vi "Packing_Barcode.vi"(7 "timeout ms":i32, 8 "error in (no error)":errorcluster, 9 "data in":string, 10 "PRINT":u16, 11 "IP":string) -> (0 "error out":errorcluster)   [LabVIEW 2017]
panel:
  # "Packing Barcode Print"
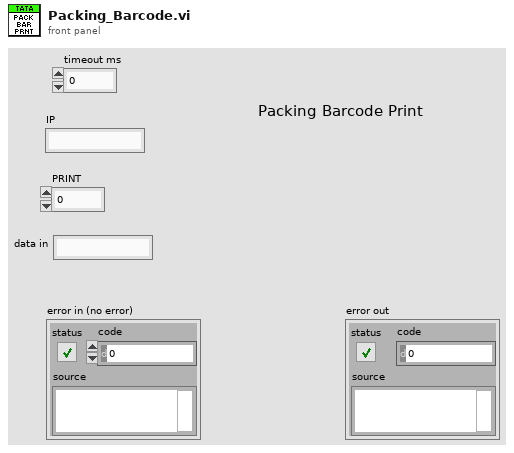
[diagram p1: front panel]
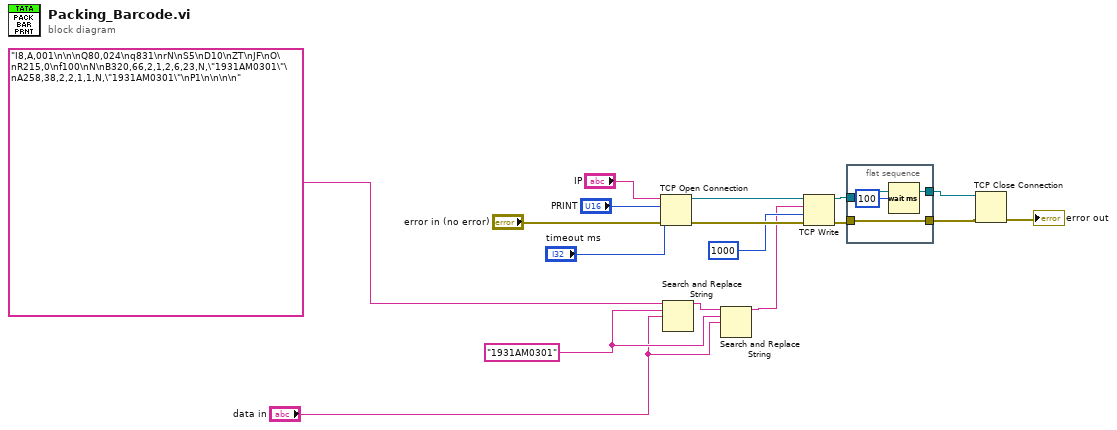
[diagram p0: block diagram]
diagram:
  w2 = "1931AM0301"
  n1 = TCP Open Connection(address="IP", remote port or service name="PRINT", timeout ms (60000)="timeout ms", error in (no error)="error in (no error)") -> (connection ID=w14:refnum<k5>, error out=w13:errorcluster)  [unwired: 1 in]
  n2 = Search and Replace String(input string="I8,A,001\n\n\nQ80,024\nq831\nrN\nS5\nD10\nZT\nJF\nO\nR215,0\nf100\nN\nB320,66,2,1,2,6,23,N,\"1931AM0301\"\nA258,38,2,2,1,1,N,\"1931AM0301\"\nP1\n\n\n\n", search string=w2, replace string="data in") -> (result string=w3:string)  [unwired: 5 in, 3 out]
  n3 = Search and Replace String(input string=w3, search string=w2, replace string="data in") -> (result string=w4:string)  [unwired: 5 in, 3 out]
  n4 = TCP Write(connection ID=w14, data in=w4, error in (no error)=w13, 9:1000 ("timeout ms (25000)")) -> (connection ID out=w15:refnum<k5>, error out=w16:errorcluster)  [unwired: 1 out]
  n5 = flat-sequence {
    tunnel: w16 -> [w19]
    tunnel: [w19] -> w10
    tunnel: w15 -> [w18]
    tunnel: [w18] -> _
    tunnel: [w18] -> w11
    frame #0 {
      n6 = Wait (ms)(milliseconds to wait=u32 100) -> ()  [unwired: 1 out]
    }
  }
  n7 = TCP Close Connection(connection ID=w11, error in (no error)=w10) -> (error out=→"error out":errorcluster)  [unwired: 1 in, 1 out]
